vi "GetEnumFeatureSymbol.vi"(9 "pFeatureName":string, 10 "handle":i64, 11 "error in (no error)":errorcluster) -> (2 "pEnumSymbol":string, 3 "error out":errorcluster)   [LabVIEW 2016]
uses:
  MVSDKmd.dll
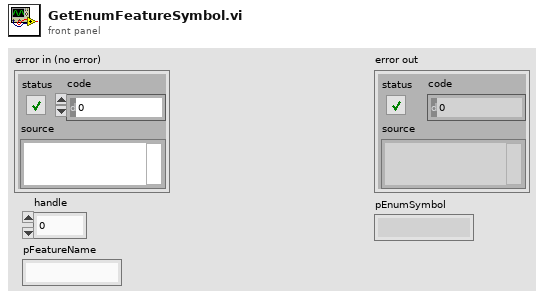
[diagram p1: front panel]
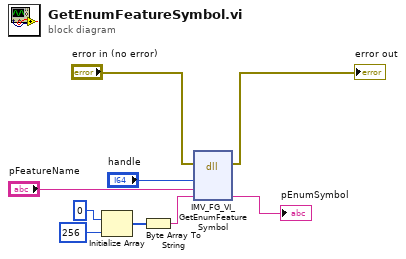
[diagram p0: block diagram]
diagram:
  n1 = Initialize Array(u8 0, 256) -> (w3:u8[])
  n2 = Byte Array To String(unsigned byte array=w3) -> (string=w2:string)
  n3 = dll-call lib="MVSDKmd.dll" fn="IMV_FG_VI_GetEnumFeatureSymbol"(error in="error in (no error)", "handle"="handle", "pFeatureName"="pFeatureName", "pEnumSymbol"=w2) -> (error out=→"error out":errorcluster, "pEnumSymbol"=→"pEnumSymbol":string)  [unwired: 5 in, 1 out]
